vi "AnMiTC_Main.vi"() -> ()   [LabVIEW 2019]
panel:
  out "T3":dbl format="%.2f"
  out "T2":dbl format="%.2f"
  in  "Tab Control":enum32{"Annealing System", "Microwave System"}(tab)
  out "T0 Chart":waveform(dbl)[](graph)
  out "T1 Chart":waveform(dbl)[](graph)
  out "T2 Chart":waveform(dbl)[](graph)
  out "T3 Chart":waveform(dbl)[](graph)
  out "status_dio":bool caption="DIO Control Status"
  in  "degC_low":dbl=5.0 caption="From"
  in  "degC_hi":dbl=45.0 caption="To"
  out "alarm_t":bool caption="Temperature Alarm"
  in  "Readout Interval":i32=5 caption="sec"
  in  "units":i32(ring) items=["degC", "degF", "kelvin", "raw"]
  out "T1":dbl format="%.2f"
  out "T0":dbl format="%.2f"
  out "Readout Status":bool
  out "Last Measured":timestamp format="%<%Y-%m-%d %H:%M:%S>T"
  in  "Stop":bool
  # "Thermocouples for Annealing & Microwave Control Systems"
  # "Annealing System"
  # "Microwave System"
  # "Good Temperature Range (degC)"
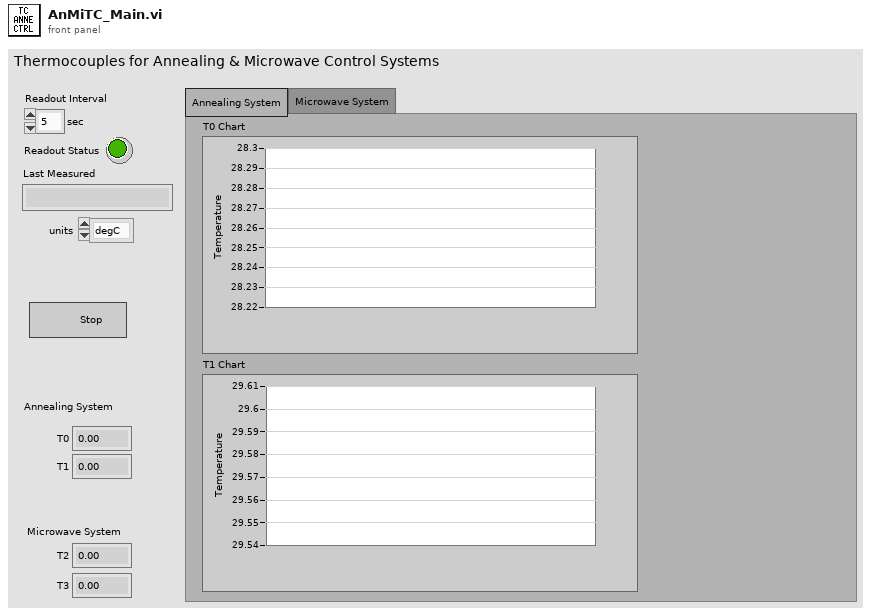
[diagram p1: front panel]
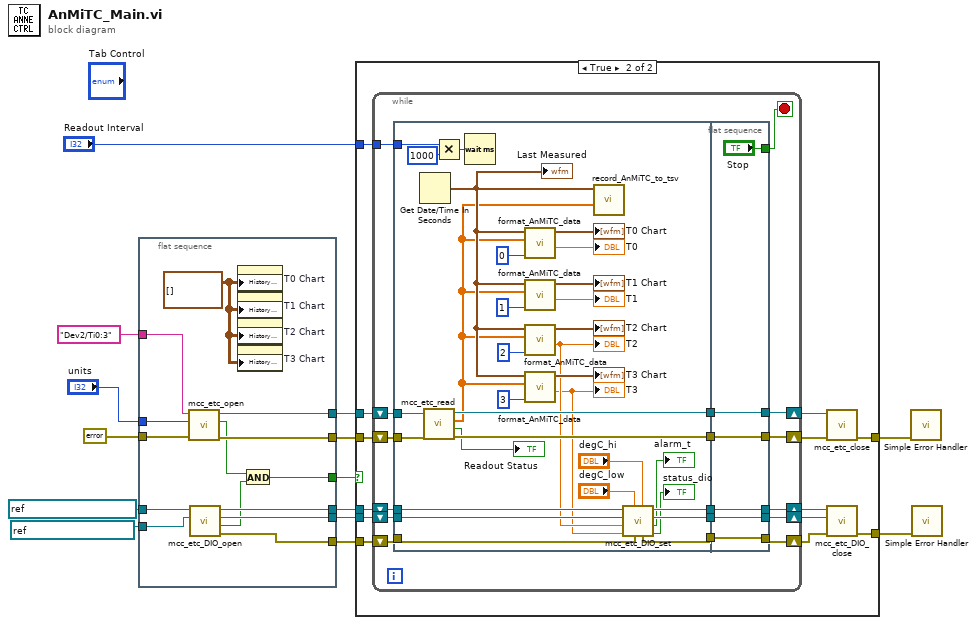
[diagram p0: block diagram]
diagram:
  n1 = flat-sequence {
    tunnel: [w28] -> w14
    tunnel: errorcluster {"status"=FALSE, "code"=0, "source"=""} ("error in") -> [w27]
    tunnel: [w26] -> w12
    tunnel: "Dev2/Ti0:3" ("Device/Channel Name") -> [w25]
    tunnel: "units" -> [w24]
    tunnel: refnum<k21> "Dev2/AuxPort/Do0" ("output_line") -> [w22]
    tunnel: refnum<k21> "Dev2/AuxPort/Di4" ("input_line") -> [w21]
    tunnel: [w20] -> w6
    tunnel: [w19] -> w5
    tunnel: [w16] -> w2
    tunnel: [w15] -> w1
    frame #0 {
      w23 = waveform(dbl)[][] [] ("History Data")
      n2 = call "mcc_etc_open.vi"("error in"=w27, "units"=w24, "name"=w25) -> ("error out"=w26:errorcluster, "status"=w18:bool, "task out"=w28:refnum<k24>)  [unwired: 6 in]
      n3 = call "mcc_etc_DIO_open.vi"("input_line"=w21, "output_line"=w22) -> ("error out"=w16:errorcluster, "status"=w17:bool, "input_task_out"=w19:refnum<k24>, "output_task out"=w20:refnum<k24>)  [unwired: 6 in]
      n4 = property on="T0 Chart" class="WFChart (strict)"("History Data"=w23) -> ()  [unwired: 2 in, 2 out]
      n5 = property on="T1 Chart" class="WFChart (strict)"("History Data"=w23) -> ()  [unwired: 2 in, 2 out]
      n6 = property on="T2 Chart" class="WFChart (strict)"("History Data"=w23) -> ()  [unwired: 2 in, 2 out]
      n7 = property on="T3 Chart" class="WFChart (strict)"("History Data"=w23) -> ()  [unwired: 2 in, 2 out]
      n8 = And(x=w18, y=w17) -> (x .and. y?=w15:bool)
    }
  }
  n9 = case shown="True" w1 {
    tunnel: w14 -> [_ w43]
    tunnel: w12 -> [w30 w42]
    tunnel: "Readout Interval" -> [_ w39]
    tunnel: w6 -> [_ w38]
    tunnel: w5 -> [_ w37]
    tunnel: [w29 w34] -> w4
    tunnel: [w30 w33] -> w3
    tunnel: w2 -> [w29 w32]
    frame False {
    }
    frame True {
      n10 = while {
        shift-right: [w58] -> w40
        shift-left: w42 -> [w59]
        shift-right: [w57] -> w41
        shift-left: w43 -> [w60]
        tunnel: w39 -> [w56]
        shift-right: [w53] -> w36
        shift-left: w38 -> [w55]
        shift-right: [w52] -> w35
        shift-left: w37 -> [w54]
        shift-right: [w50] -> w31
        shift-left: w32 -> [w51]
        stop <- w44 stop-if-true
        n11 = flat-sequence {
          tunnel: w60 -> [w92]
          tunnel: w59 -> [w91]
          tunnel: w56 -> [w87]
          tunnel: w55 -> [w82]
          tunnel: w54 -> [w81]
          tunnel: w51 -> [w78]
          tunnel: [w90] -> w49
          tunnel: [w89] -> w48
          tunnel: [w80] -> w47
          tunnel: [w79] -> w46
          tunnel: [w77] -> w45
          tunnel: [w94] -> w50
          tunnel: [w95] -> w52
          tunnel: [w96] -> w53
          tunnel: [w97] -> w57
          tunnel: [w98] -> w58
          tunnel: w49 -> [w98]
          tunnel: w48 -> [w97]
          tunnel: w47 -> [w96]
          tunnel: w46 -> [w95]
          tunnel: w45 -> [w94]
          tunnel: ["Stop"] -> w44
          frame #0 {
            n12 = Get Date/Time In Seconds() -> (seconds since 1Jan1904=w72:timestamp)
            "Last Measured" <- w72
            n13 = call "mcc_etc_read.vi"("error in"=w91, "task in"=w92) -> ("error out"=w90:errorcluster, "status"=→"Readout Status":bool, "temperature_array"=w65:dbl[], "task out"=w89:refnum<k24>)  [unwired: 6 in]
            n14 = Multiply(x=w87, y=1000) -> (x*y=w62:i32)
            n15 = Wait (ms)(milliseconds to wait=w62) -> ()  [unwired: 1 out]
            n16 = call "format_AnMiTC_data.vi"("index"=0, "value_array"=w65, "time"=w72) -> ("value"=→"T0":dbl, "waveform_array"=→"T0 Chart":waveform(dbl)[])  [unwired: 7 in]
            n17 = call "format_AnMiTC_data.vi"("index"=1, "value_array"=w65, "time"=w72) -> ("value"=→"T1":dbl, "waveform_array"=→"T1 Chart":waveform(dbl)[])  [unwired: 7 in]
            n18 = call "format_AnMiTC_data.vi"("index"=2, "value_array"=w65, "time"=w72) -> ("value"=w64:dbl, "waveform_array"=→"T2 Chart":waveform(dbl)[])  [unwired: 7 in]
            "T2" <- w64
            n19 = call "format_AnMiTC_data.vi"("index"=3, "value_array"=w65, "time"=w72) -> ("value"=w63:dbl, "waveform_array"=→"T3 Chart":waveform(dbl)[])  [unwired: 7 in]
            "T3" <- w63
            n20 = call "record_AnMiTC_to_tsv.vi"("temperatures"=w65, "time"=w72) -> ()  [unwired: 10 in]
            n21 = call "mcc_etc_DIO_set.vi"("degC_hi"="degC_hi", "error in"=w78, "degC_low"="degC_low", "degC_ch2"=w63, "degC_ch1"=w64, "input_line"=w81, "output_line"=w82) -> ("DIO_control_status"=→"status_dio":bool, "alarm"=→"alarm_t":bool, "input_line_out"=w79:refnum<k24>, "output_line_out"=w80:refnum<k24>, "error out"=w77:errorcluster)
          }
          frame #1 {
          }
        }
      }
      n22 = call "mcc_etc_close.vi"("error in"=w40, "task in"=w41) -> ("error out"=w33:errorcluster)  [unwired: 8 in, 1 out]
      n23 = call "mcc_etc_DIO_close.vi"("error in"=w31, "input_line"=w35, "output_line"=w36) -> ("error out"=w34:errorcluster)  [unwired: 8 in]
    }
  }
  n24 = call <vilib>:"Simple Error Handler.vi"("error in (no error)"=w3) -> ()  [unwired: 4 in, 5 out]
  n25 = call <vilib>:"Simple Error Handler.vi"("error in (no error)"=w4) -> ()  [unwired: 4 in, 5 out]
